vi "Z900_navX_SERIAL_CapturePacket.vi"(11 "Buffer":string) -> (0 "Packet Size":i32, 1 "Packet Located":bool, 2 "Packet":string, 3 "Buffer":string)   [LabVIEW 2015, in "navX Library v2.lvlib"]
uses:
  navX Library v2.lvlib
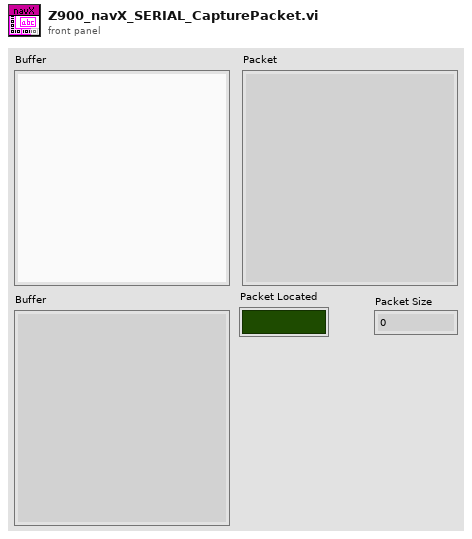
[diagram p1: front panel]
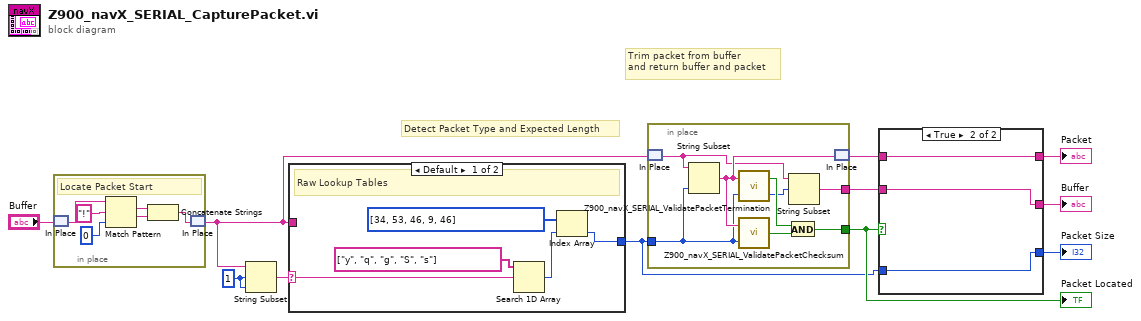
[diagram p0: block diagram]
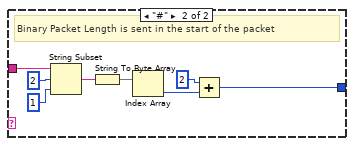
[diagram p2: hidden frame]
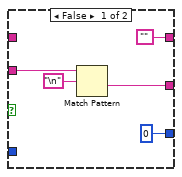
[diagram p3: hidden frame]
diagram:
  w3 = 1 ("length (rest)")
  # "Trim packet from buffer\nand return buffer and packet"
  # "Detect Packet Type and Expected Length"
  n1 = in-place {
    # "Locate Packet Start"
    n2 = in-place-match #1("Buffer") -> (w14:string)
    n3 = Match Pattern(string=w14, regular expression="!" ("Packet Start Char"), offset (0)=0 ("offset past match")) -> (match substring=w17:string, after substring=w16:string)  [unwired: 2 out]
    n4 = Concatenate Strings(w17, w16) -> (w13:string)
    n5 = in-place-match #1(w13) -> (w10:string)
  }
  n6 = String Subset(string=w10, offset (0)=w3, length (rest)=w3) -> (substring=w2:string)
  n7 = case shown="Default" w2 {
    selector: w2 -> [w18 _]
    tunnel: [w19 w26] -> w4
    tunnel: w10 -> [_ w24]
    frame Default {
      # "Raw Lookup Tables"
      n8 = Search 1D Array(1D array=string[] ["y", "q", "g", "S", "s"], element=w18) -> (index of element=w20:i32)  [unwired: 1 in]
      n9 = Index Array(array=i32[] [34, 53, 46, 9, 46], index=w20) -> (element=w19:i32)
    }
    frame "#" {
      # "Binary Packet Length is sent in the start of the packet"
      n10 = String Subset(string=w24, offset (0)=2, length (rest)=1 ("length (rest)")) -> (substring=w25:string)
      n11 = String To Byte Array(string=w25) -> (unsigned byte array=w28:u8[])
      n12 = Index Array(array=w28) -> (element=w29:u8)  [unwired: 1 in]
      n13 = Add(x=u8 2 ("y"), y=w29) -> (x+y=w26:u8)
    }
  }
  n14 = in-place {
    in-place-border: w4 -> [w37]
    in-place-border: [w34] -> w9
    in-place-border: [w31] -> w1
    n15 = in-place-match #2(w10) -> (w32:string)
    n16 = String Subset(string=w32, length (rest)=w37) -> (substring=w38:string)  [unwired: 1 in]
    n17 = call "Z900_navX_SERIAL_ValidatePacketTermination.vi"("Expected Packet Length"=w37, "Buffer"=w38) -> ("Packet Termination Offset"=w33:i32, "Packet Valid"=w35:bool)
    n18 = call "Z900_navX_SERIAL_ValidatePacketChecksum.vi"("Expected Packet Length"=w37, "Buffer"=w38) -> ("Packet Valid"=w36:bool)
    n19 = And(x=w35, y=w36) -> (x .and. y?=w34:bool)
    n20 = String Subset(string=w32, offset (0)=w33) -> (substring=w31:string)  [unwired: 1 in]
    n21 = in-place-match #2(w38) -> (w7:string)
  }
  "Packet Located" <- w9
  n22 = case shown="True" w9 {
    tunnel: ["" w46] -> w8
    tunnel: w7 -> [_ w46]
    tunnel: [w40 w45] -> w6
    tunnel: w1 -> [w42 w45]
    tunnel: [0 w44] -> w5
    tunnel: w4 -> [_ w44]
    frame False {
      n23 = Match Pattern(string=w42, regular expression="\n") -> (after substring=w40:string)  [unwired: 1 in, 3 out]
    }
    frame True {
    }
  }
  "Packet" <- w8
  "Buffer" <- w6
  "Packet Size" <- w5
